vi "Plot GPS Logfile.vi"(1 "file path (dialog if empty)":path=path "C:/Users/ATV Project/Dropbox/Auto-Steering and Obstacle Avoidance System Project/Software/VI's/_Data/Log_Files(GPS)/GPS_LOG_5-6-2013_6-12 PM") -> (0 "Navigation Duration(s)":i32)   [LabVIEW 2011]
uses:
  <vilib>/Utility/file.llb/Read From Spreadsheet File (DBL).vi
  _GlobalVariables&Libraries/ATV Program Global Variables.vi
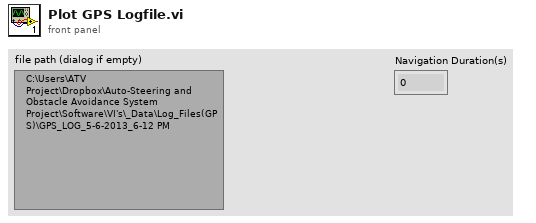
[diagram p1: front panel]
types:
  T1 = cluster{"Navigation Coordinates":cluster{"Latitude":dbl, "Longitude":dbl}[], "Coordinate Count":u32, "Drive Speed":string, "Steer Angle":dbl, "Steering":dbl, "Direction to next Coordinate":dbl, "Drive":dbl, "Navigation Path":string}
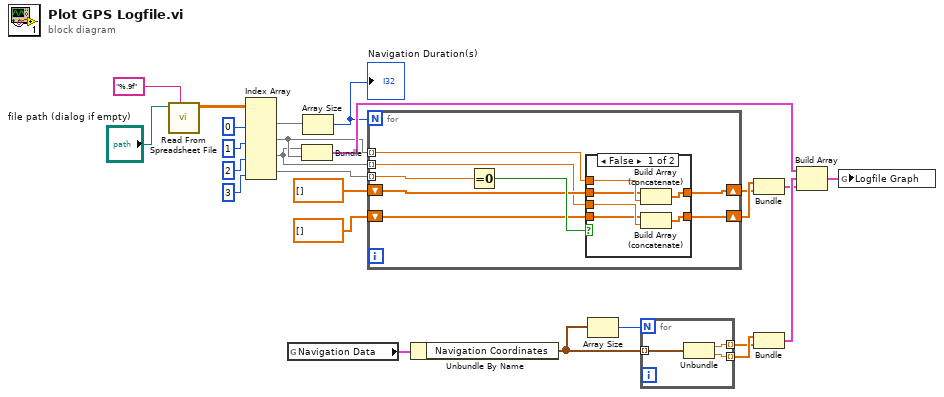
[diagram p0: block diagram]
diagram:
  n1 = call-poly <vilib>:"Read From Spreadsheet File.vi"("format (%.3f)"="%.9f", "file path (dialog if empty)"="file path (dialog if empty)") -> ("all rows"=w12:dbl[][])  [unwired: 5 in, 4 out]
  n2 = Index Array(array=w12, index (col) #1=0 ("disabled index (col)"), index (col) #2=1 ("index (col)"), index (col) #3=2 ("index (col)"), index (col) #4=3 ("index (col)")) -> (element #1=w11:dbl[], element #2=w7:dbl[], element #3=w6:dbl[], element #4=w8:dbl[])  [unwired: 4 in]
  n3 = global read "ATV Program Global Variables.vi" "Navigation Data"() -> (w24:T1)
  n4 = Bundle("all rows"=w6, "all rows"=w7) -> (w14:cluster{"all rows":dbl[], "all rows":dbl[]})  [unwired: 1 in]
  n5 = Array Size(array=w11) -> (size(s)=w9:i32)
  "Navigation Duration(s)" <- w9
  n6 = for {
    N: w9 -> [_]
    tunnel: w8 -> [w33] mode=indexing
    tunnel: w7 -> [w28] mode=indexing
    tunnel: w6 -> [w29] mode=indexing
    shift-right: [w31] -> w3
    shift-left: dbl[] [] -> [w30]
    shift-right: [w27] -> w4
    shift-left: dbl[] [] -> [w26]
    n7 = Equal To 0?(x=w33) -> (x = 0?=w32:bool)
    n8 = case shown="False" w32 {
      tunnel: [w37 w41] -> w31
      tunnel: w30 -> [w34 w41]
      tunnel: w29 -> [w38 _]
      tunnel: w28 -> [w39 _]
      tunnel: [w36 w40] -> w27
      tunnel: w26 -> [w35 w40]
      frame False {
        n9 = Build Array (concatenate)(w34, w39) -> (w37:dbl[])
        n10 = Build Array (concatenate)(w35, w38) -> (w36:dbl[])
      }
      frame True {
      }
    }
  }
  n11 = Unbundle By Name(w24) -> ("Navigation Coordinates"=w22:cluster{"Latitude":dbl, "Longitude":dbl}[])
  n12 = Array Size(array=w22) -> (size(s)=w23:i32)
  n13 = for {
    N: w23 -> [_]
    tunnel: w22 -> [w44] mode=indexing
    tunnel: [w43] -> w20 mode=indexing
    tunnel: [w42] -> w21 mode=indexing
    n14 = Unbundle(w44) -> ("Latitude"=w43:dbl, "Longitude"=w42:dbl)
  }
  n15 = Bundle(w4, w3) -> (w5:cluster{dbl[], dbl[]})  [unwired: 1 in]
  n16 = Bundle(w21, w20) -> (w19:cluster{dbl[], dbl[]})  [unwired: 1 in]
  n17 = Build Array(w14, w19, w5) -> (w13:cluster{"all rows":dbl[], "all rows":dbl[]}[])
  n18 = global write "ATV Program Global Variables.vi" "Logfile Graph"(w13) -> ()
